vi "channelSelected.vi"(8 "error in (no error)":errorcluster, 11 "StaticOutputEditor in":refnum<class "StaticOutputEditor.lvclass">) -> (0 "error out":errorcluster, 3 "StaticOutputEditor out":refnum<class "StaticOutputEditor.lvclass">)   [LabVIEW 2011, in "Views.lvlib" / "ScriptEditor.lvlib" / "StaticOutputEditor.lvclass"]
uses:
  StaticOutputEditor.lvclass
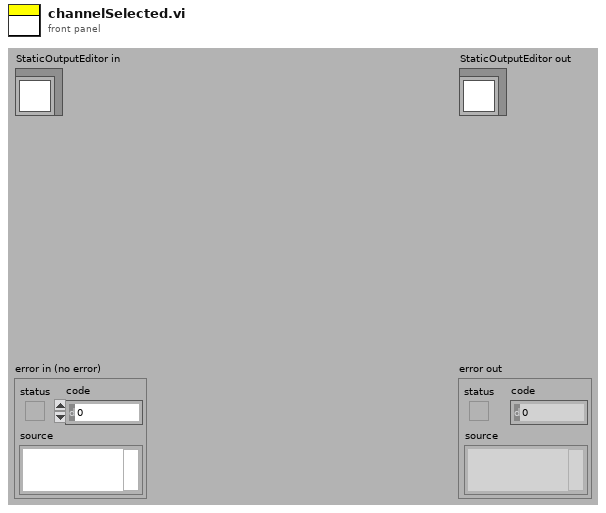
[diagram p1: front panel]
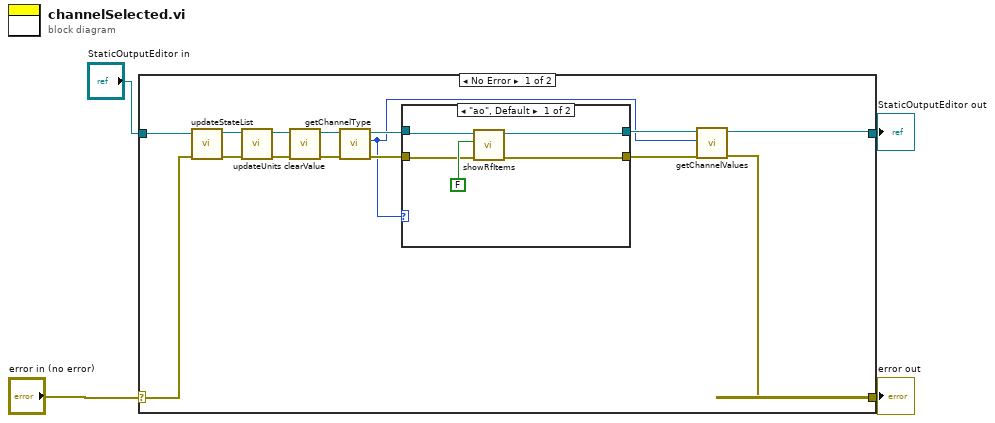
[diagram p0: block diagram]
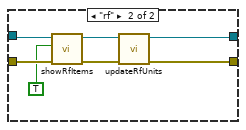
[diagram p2: hidden frame]
diagram:
  n1 = case shown="No Error" "error in (no error)" {
    selector: "error in (no error)" -> [w14 w33]
    tunnel: [w5 w33] -> w3
    tunnel: [w8 w32] -> w1
    tunnel: "StaticOutputEditor in" -> [w15 w32]
    frame No Error {
      n2 = call "updateStateList.vi"("error in (no error)"=w14, "StaticOutputEditor in"=w15) -> ("error out"=w18:errorcluster, "StaticOutputEditor out"=w19:refnum<class "StaticOutputEditor.lvclass">)  [unwired: 8 in]
      n3 = call "updateUnits.vi"("error in (no error)"=w18, "StaticOutputEditor in"=w19) -> ("error out"=w16:errorcluster, "StaticOutputEditor out"=w17:refnum<class "StaticOutputEditor.lvclass">)  [unwired: 8 in]
      n4 = call "clearValue.vi"("error in (no error)"=w16, "StaticOutputEditor in"=w17) -> ("error out"=w12:errorcluster, "StaticOutputEditor out"=w13:refnum<class "StaticOutputEditor.lvclass">)  [unwired: 8 in]
      n5 = call "getChannelType.vi"("error in (no error)"=w12, "StaticOutputEditor in"=w13) -> ("error out"=w10:errorcluster, "channel_type"=w7:enum16{"ao", "do", "ai", "di", "rf"}, "StaticOutputEditor out"=w11:refnum<class "StaticOutputEditor.lvclass">)  [unwired: 7 in]
      n6 = case shown="\"ao\", Default" w7 {
        tunnel: w11 -> [w23 w31]
        tunnel: w10 -> [w22 w30]
        tunnel: [w21 w27] -> w6
        tunnel: [w20 w25] -> w9
        frame "ao", Default {
          n7 = call "showRfItems.vi"("error in (no error)"=w22, "show/hide"=FALSE, "StaticOutputEditor in"=w23) -> ("error out"=w21:errorcluster, "StaticOutputEditor out"=w20:refnum<class "StaticOutputEditor.lvclass">)  [unwired: 7 in]
        }
        frame "rf" {
          n8 = call "showRfItems.vi"("error in (no error)"=w30, "show/hide"=TRUE, "StaticOutputEditor in"=w31) -> ("error out"=w26:errorcluster, "StaticOutputEditor out"=w28:refnum<class "StaticOutputEditor.lvclass">)  [unwired: 7 in]
          n9 = call "updateRfUnits.vi"("error in (no error)"=w26, "StaticOutputEditor in"=w28) -> ("error out"=w27:errorcluster, "StaticOutputEditor out"=w25:refnum<class "StaticOutputEditor.lvclass">)  [unwired: 8 in]
        }
      }
      n10 = call "getChannelValues.vi"("error in (no error)"=w6, "channel_type"=w7, "StaticOutputEditor in"=w9) -> ("error out"=w5:errorcluster, "StaticOutputEditor out"=w8:refnum<class "StaticOutputEditor.lvclass">)  [unwired: 7 in]
    }
    frame Error {
    }
  }
  "error out" <- w3
  "StaticOutputEditor out" <- w1
